vi "Set Para.vi"(0 "reference in":refnum<class "Context.lvclass">, 1 "Operation.lvclass":refnum<class "Operation.lvclass">, 2 "X":dbl, 4 "Y":dbl, 5 "error in (no error)":errorcluster) -> (14 "reference out":refnum<class "Context.lvclass">, 15 "result":dbl, 19 "error out":errorcluster)   [LabVIEW 2013, in "Context.lvclass"]
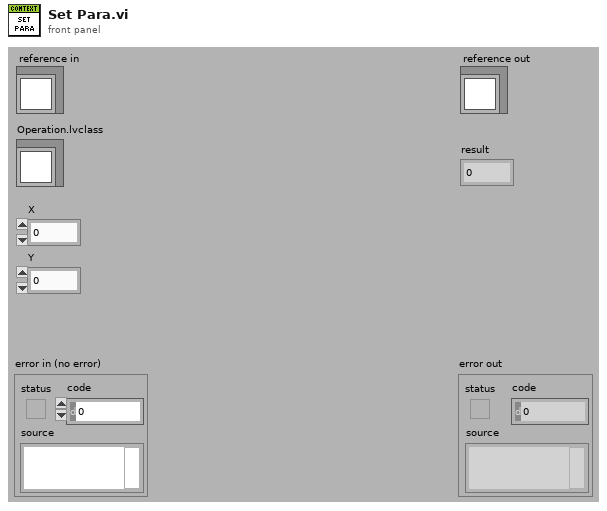
[diagram p1: front panel]
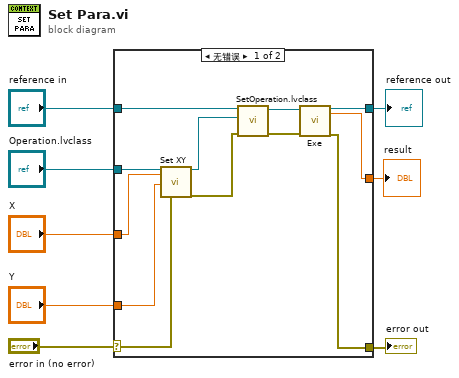
[diagram p0: block diagram]
diagram:
  n1 = case shown="无错误" "error in (no error)" {
    selector: "error in (no error)" -> [w15 w22]
    tunnel: [w10 w22] -> w7
    tunnel: [w11 w21] -> w5
    tunnel: "reference in" -> [w20 w21]
    tunnel: "Operation.lvclass" -> [w19 _]
    tunnel: "X" -> [w18 _]
    tunnel: "Y" -> [w17 _]
    tunnel: [w9 _] -> w1
    frame No Error {
      n2 = call-dynamic "Set XY.vi"("reference in"=w19, "x"=w18, "y"=w17, "error in (no error)"=w15) -> ("reference out"=w16:refnum<class "Operation.lvclass">, "error out"=w14:errorcluster)  [unwired: 14 in]
      n3 = call "SetOperation.lvclass.vi"("error in (no error)"=w14, "Operation.lvclass"=w16, "reference in"=w20) -> ("error out"=w12:errorcluster, "reference out"=w13:refnum<class "Context.lvclass">)  [unwired: 7 in]
      n4 = call-dynamic "Exe.vi"("reference in"=w13, "error in (no error)"=w12) -> ("reference out"=w11:refnum<class "Context.lvclass">, "result"=w9:dbl, "error out"=w10:errorcluster)  [unwired: 15 in]
    }
    frame Error {
    }
  }
  "error out" <- w7
  "reference out" <- w5
  "result" <- w1
